vi "Legend VI.vi"() -> (0 "Array":cluster{"Color Box":u32, "String":string}[][](array[cluster])=[[{"Color Box"=16750899, "String"="In Work (Answer Today)"}, {"Color Box"=14417800, "String"="In Work"}, {"Color Box"=16737945, "String"="In Collab (Answer Today)"}, {"Color Box"=6737151, "String"="In Collab"}, {"Color Box"=4713287, "String"=""}, {"Color Box"=9746580, "String"=""}, {"Color Box"=16580608, "String"=""}]])   [LabVIEW 2018]
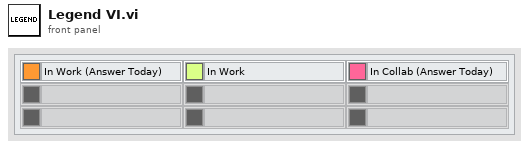
[diagram p1: front panel]
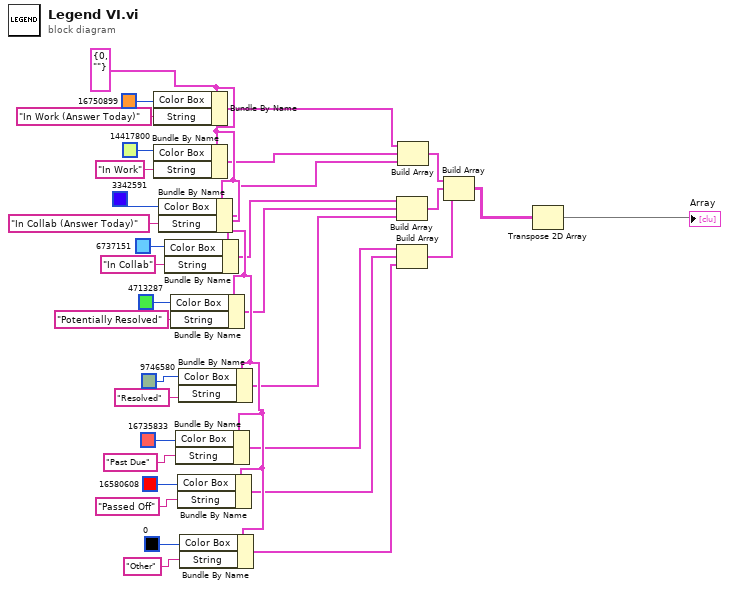
[diagram p0: block diagram]
diagram:
  w12 = cluster{"Color Box":u32, "String":string} {"Color Box"=0, "String"=""} ("element")
  n1 = Bundle By Name(cluster=w12, "Color Box"=u32 16750899, "String"="In Work (Answer Today)") -> (w2:cluster{"Color Box":u32, "String":string})
  n2 = Bundle By Name(cluster=w12, "Color Box"=u32 14417800, "String"="In Work") -> (w3:cluster{"Color Box":u32, "String":string})
  n3 = Bundle By Name(cluster=w12, "Color Box"=u32 3342591, "String"="In Collab (Answer Today)") -> (w4:cluster{"Color Box":u32, "String":string})
  n4 = Bundle By Name(cluster=w12, "Color Box"=u32 6737151, "String"="In Collab") -> (w5:cluster{"Color Box":u32, "String":string})
  n5 = Bundle By Name(cluster=w12, "Color Box"=u32 4713287, "String"="Potentially Resolved") -> (w6:cluster{"Color Box":u32, "String":string})
  n6 = Bundle By Name(cluster=w12, "Color Box"=u32 16735833, "String"="Past Due") -> (w8:cluster{"Color Box":u32, "String":string})
  n7 = Bundle By Name(cluster=w12, "Color Box"=u32 16580608, "String"="Passed Off") -> (w9:cluster{"Color Box":u32, "String":string})
  n8 = Bundle By Name(cluster=w12, "Color Box"=u32 9746580, "String"="Resolved") -> (w7:cluster{"Color Box":u32, "String":string})
  n9 = Bundle By Name(cluster=w12, "Color Box"=u32 0, "String"="Other") -> (w10:cluster{"Color Box":u32, "String":string})
  n10 = Build Array(w5, w6, w7) -> (w11:cluster{"Color Box":u32, "String":string}[])
  n11 = Build Array(w8, w9, w10) -> (w1:cluster{"Color Box":u32, "String":string}[])
  n12 = Build Array(w2, w3, w4) -> (w19:cluster{"Color Box":u32, "String":string}[])
  n13 = Build Array(w19, w11, w1) -> (w18:cluster{"Color Box":u32, "String":string}[][])
  n14 = Transpose 2D Array(2D array=w18) -> (transposed array=→"Array":cluster{"Color Box":u32, "String":string}[][])
